vi "Modbus Request.vi"(0 "TCP Network Connection in":refnum<k5>, 1 "Function Codes":T1 items=["Read Coil Status"=1, "Read Input Status"=2, "Read Holding Registers"=3, "Read Input Registers"=4, "Force Single Coil"=5, "Preset Single Register"=6, "Force Multiple Coils"=15, "Preset Multiple Registers"=16], 2 "Start Address":u16, 3 "Payload":string, 5 "error in (no error)":errorcluster, 9 "timeout ms (1000)":i32=1000) -> (14 "TCP Network Connection out":refnum<k5>, 15 "Payload":string, 16 "MBAP":T3, 17 "Response PDU":T4, 18 "Exception":T2, 19 "error out":errorcluster)   [LabVIEW 2023, in "Modbus TCP Micro.lvlib"]
uses:
  Modbus TCP Micro.lvlib
  Response PDU.ctl
  MBAP Header.ctl
  Modbus Exception.ctl
  Modbus Functions.ctl
  Modbus Request.ctl
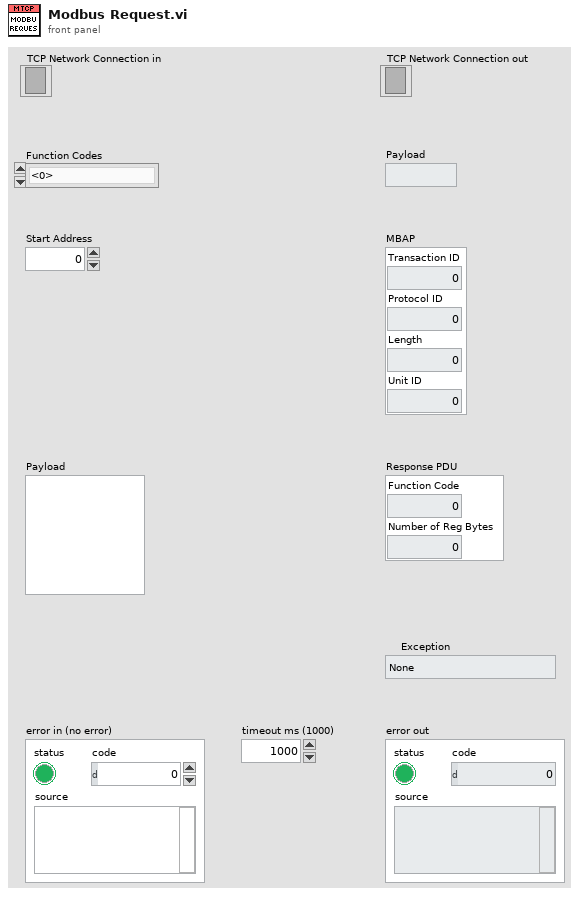
[diagram p1: front panel]
types:
  T1 = typedef "Modbus TCP Micro.lvlib/Modbus Functions.ctl" = u8
  T2 = typedef "Modbus TCP Micro.lvlib/Modbus Exception.ctl" = enum16{"None", "Illegal Function", "Illegal Data Address", "Illegal Data Value", "Slave Device Failure", "ACK", "Slave Device Busy", "NACK", "Memory Parity Error", "Unknown", "Gateway Path Unavailable", "Gateway Target Device Failed to Respond"}
  T3 = typedef "Modbus TCP Micro.lvlib/MBAP Header.ctl" = cluster{"Transaction ID":u16, "Protocol ID":u16, "Length":u16, "Unit ID":u8}
  T4 = typedef "Modbus TCP Micro.lvlib/Response PDU.ctl" = cluster{"Function Code":u8, "Number of Reg Bytes":u8}
  T5 = typedef "Modbus TCP Micro.lvlib/Modbus Request.ctl" = cluster{"Function Code":u8, "Start Address":u16}
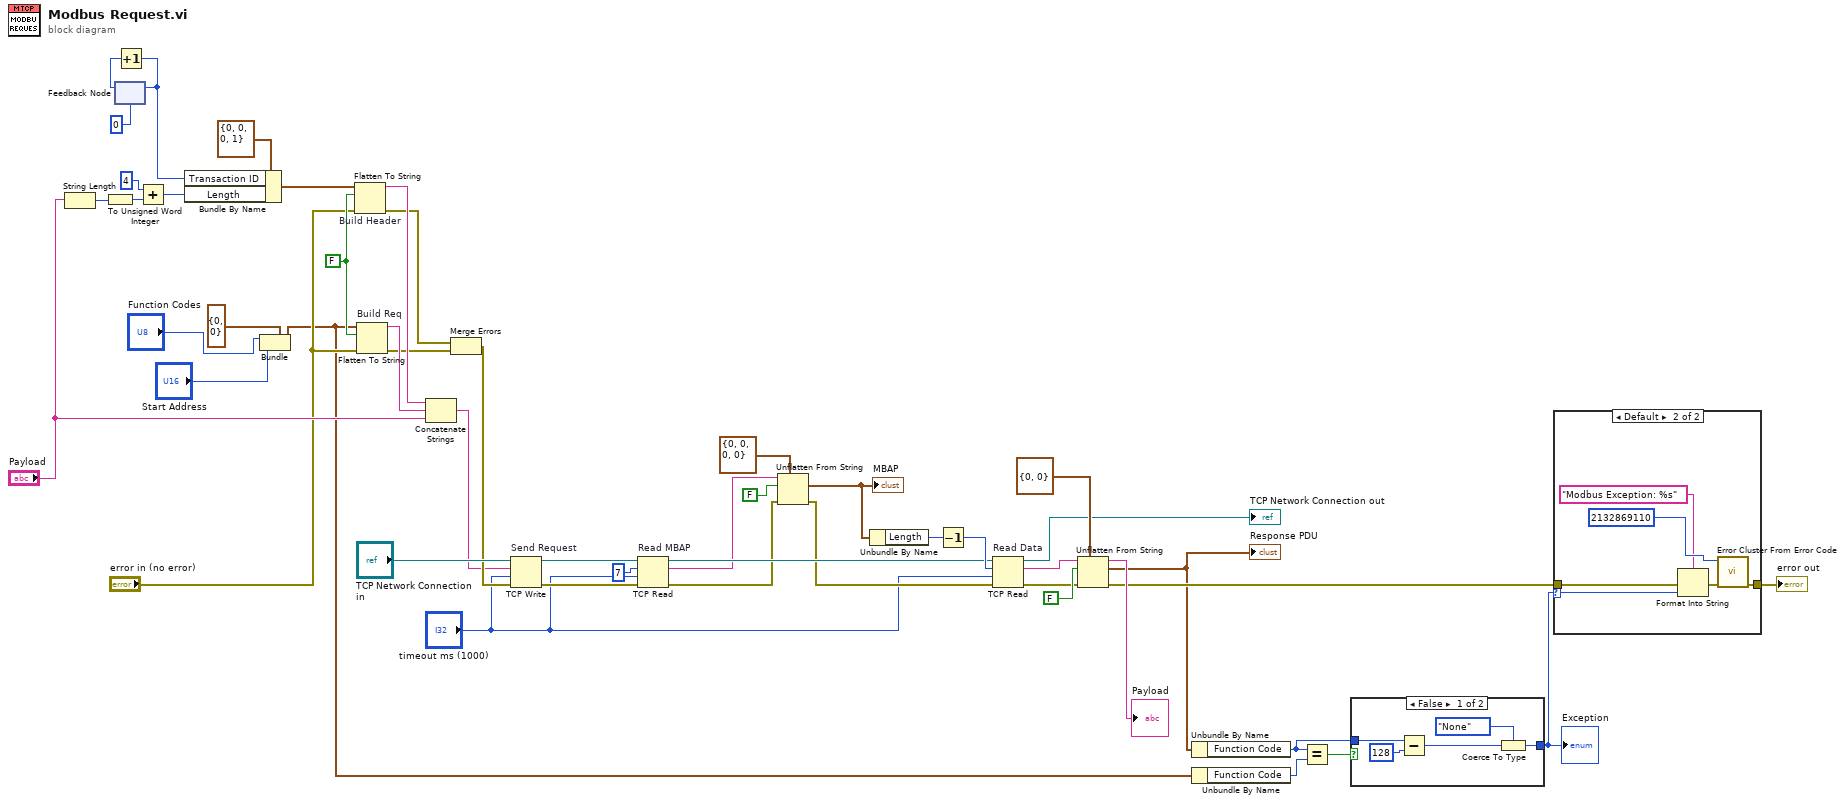
[diagram p0: block diagram]
diagram:
  w48 = FALSE ("prepend array or string size? (T)")
  n1 = String Length(string="Payload") -> (length=w25:i32)
  n2 = To Unsigned Word Integer(number=w25) -> (unsigned 16bit integer=w24:u16)
  n3 = feedback #1(u16 0) -> (w10:u16)
  n4 = Increment(x=w10) -> (x+1=w9:u16)
  n5 = feedback-in #1(w9) -> ()
  n6 = Add(x=u16 4 ("Length"), y=w24) -> (x+y=w26:u16)
  n7 = Bundle By Name(cluster=T3 {"Transaction ID"=0, "Protocol ID"=0, "Length"=0, "Unit ID"=1} ("MBAP in"), "Transaction ID"=w9, "Length"=w26) -> (w29:T3)
  n8 = Bundle(cluster=T5 {"Function Code"=0, "Start Address"=0} ("Request"), "Function Code"="Function Codes", "Start Address"="Start Address") -> (w5:T5)
  n9 = Flatten To String "Build Header"(anything=w29, prepend array or string size? (T)=w48, error in (no error)="error in (no error)") -> (data string=w35:string, error out=w11:errorcluster)  [unwired: 1 in, 1 out]
  n10 = Flatten To String "Build Req"(anything=w5, prepend array or string size? (T)=w48, error in (no error)="error in (no error)") -> (data string=w49:string, error out=w23:errorcluster)  [unwired: 1 in, 1 out]
  n11 = Concatenate Strings(w35, w49, "Payload") -> (w7:string)
  n12 = Merge Errors(w11, w23) -> (w12:errorcluster)
  n13 = TCP Write "Send Request"(connection ID="TCP Network Connection in", data in=w7, error in (no error)=w12, 9:"timeout ms (1000)") -> (connection ID out=w33:refnum<k5>, error out=w31:errorcluster)  [unwired: 1 out]
  n14 = TCP Read "Read MBAP"(connection ID=w33, bytes to read=7, error in (no error)=w31, 9:"timeout ms (1000)") -> (connection ID out=w40:refnum<k5>, data out=w38:string, error out=w22:errorcluster)  [unwired: 1 in]
  n15 = Unflatten From String(type=T3 {"Transaction ID"=0, "Protocol ID"=0, "Length"=0, "Unit ID"=0}, binary string=w38, data includes array or string size? (T)=FALSE, error in (no error)=w22) -> (value=w45:T3, error out=w21:errorcluster)  [unwired: 1 in, 1 out]
  "MBAP" <- w45
  n16 = Unbundle By Name(w45) -> ("Length"=w41:u16)
  n17 = Decrement(x=w41) -> (x-1=w47:u16)
  n18 = TCP Read "Read Data"(connection ID=w40, bytes to read=w47, error in (no error)=w21, 9:"timeout ms (1000)") -> (connection ID out=→"TCP Network Connection out":refnum<k5>, data out=w43:string, error out=w20:errorcluster)  [unwired: 1 in]
  n19 = Unflatten From String(type=T4 {"Function Code"=0, "Number of Reg Bytes"=0}, binary string=w43, data includes array or string size? (T)=FALSE, error in (no error)=w20) -> (rest of the binary string=→"Payload":string, value=w18:T4, error out=w19:errorcluster)  [unwired: 1 in]
  "Response PDU" <- w18
  n20 = Unbundle By Name(w18) -> ("Function Code"=w17:u8)
  n21 = Unbundle By Name(w5) -> ("Function Code"=w15:u8)
  n22 = Equal?(x=w17, y=w15) -> (x = y?=w14:bool)
  n23 = case shown="False" w14 {
    tunnel: [w51 _] -> w1
    tunnel: w17 -> [w50 _]
    frame False {
      n24 = Subtract(x=w50, y=u8 128) -> (x-y=w52:u8)
      n25 = Coerce To Type(0:w52, 1:Modbus_Exception."None") -> (2:w51:T2)
    }
    frame True {
    }
  }
  "Exception" <- w1
  n26 = case shown="Default" w1 {
    selector: w1 -> [_ w57]
    tunnel: w19 -> [w55 w61]
    tunnel: [w55 w60] -> w2
    frame "None" {
    }
    frame Default {
      n27 = Format Into String(format string="Modbus Exception: %s", error in=w61, w57) -> (error out=w58:errorcluster)  [unwired: 1 in, 1 out]
      n28 = call <vilib>:"Error Cluster From Error Code.vi"("error in (no error)"=w58, "error code (0)"=2132869110) -> ("error out"=w60:errorcluster)  [unwired: 7 in]
    }
  }
  "error out" <- w2
